vi "QTrkTest.vi"() -> ()   [LabVIEW 2011]
uses:
  QTrk.llb/QTrkSettings.ctl
panel:
  in  "Select dll":bool
  out "Sample img":sgl[][](graph)
  in  "stop test":bool
  out "Frame#":i32
  out "Frames/s":dbl
  in  "Testing sample count":i32=10000
  out "testing results":i32
  out "Single ZLUT plane image":sgl[][](graph)
  in  "Run":bool
  in  "stop":bool
  in  "LUT radii":cluster{"min":sgl, "max":sgl}={"min"=0.0, "max"=40.0}
  out "LUT":u8[][](graph)
  out "zlut results":i32
  out "Generated LUT":sgl[][](graph)
  in  "Max Z":dbl=180.0
  in  "Min Z":dbl
  in  "QTrk Settings":T1={"Image width"=150, "Image height"=150, "Number of threads (CPU based)"=-1, "Max Queue Size"=128, "XCOR Profile Length"=32, "XCOR Profile Width"=2, "XCOR Iterations"=5, "ZLUT MinRadius"=5.0, "ZLUT MaxRadius"=60.0, "ZLUT AngularSteps"=128, "QI Iterations"=4, "QI RadialSteps"=64, "QI AngularSteps Per Quadrant"=32, "QI MinRadius"=2.0, "QI MaxRadius"=60.0, "CUDA Device# (if using cuda)"=0, "COM Background correction factor"=2.0, "ZLUT RadialSteps"=64, "Gaussian 2D Fit Iterations"=8}
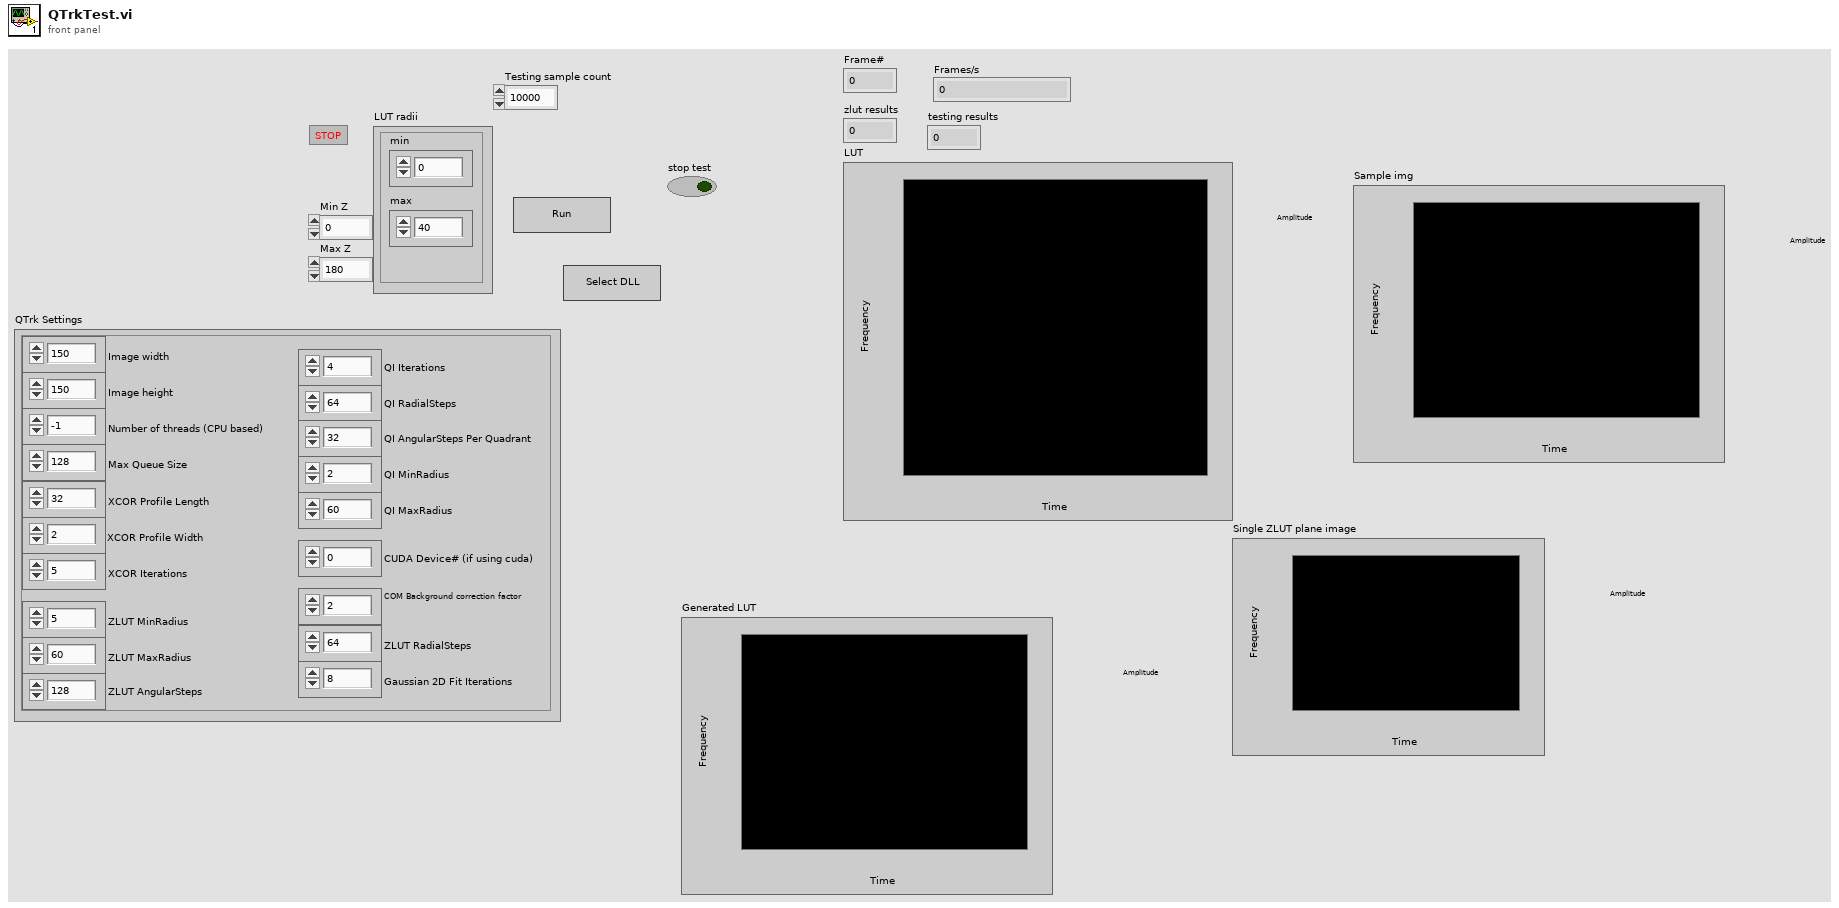
[diagram p1: front panel]
types:
  T1 = typedef "QTrkSettings.ctl" = cluster{"Image width":i32, "Image height":i32, "Number of threads (CPU based)":i32, "Max Queue Size":i32, "XCOR Profile Length":i32, "XCOR Profile Width":i32, "XCOR Iterations":i32, "ZLUT MinRadius":sgl, "ZLUT MaxRadius":sgl, "ZLUT AngularSteps":i32, "QI Iterations":i32, "QI RadialSteps":i32, "QI AngularSteps Per Quadrant":i32, "QI MinRadius":sgl, "QI MaxRadius":sgl, "CUDA Device# (if using cuda)":i32, "COM Background correction factor":sgl, "ZLUT RadialSteps":i32, "Gaussian 2D Fit Iterations":i32}
  T2 = typedef "Image Type" = u32
  T3 = typedef "IMAQ Image.ctl" = refnum<image>
  T4 = enum16{"Center-of-Mass", "1D Cross-Correlation", "Quadrant Interpolation"}
  T5 = typedef "QTrkInstance.ctl" = cluster{"QTrk Pointer":u64, "QTrk Settings":T1}
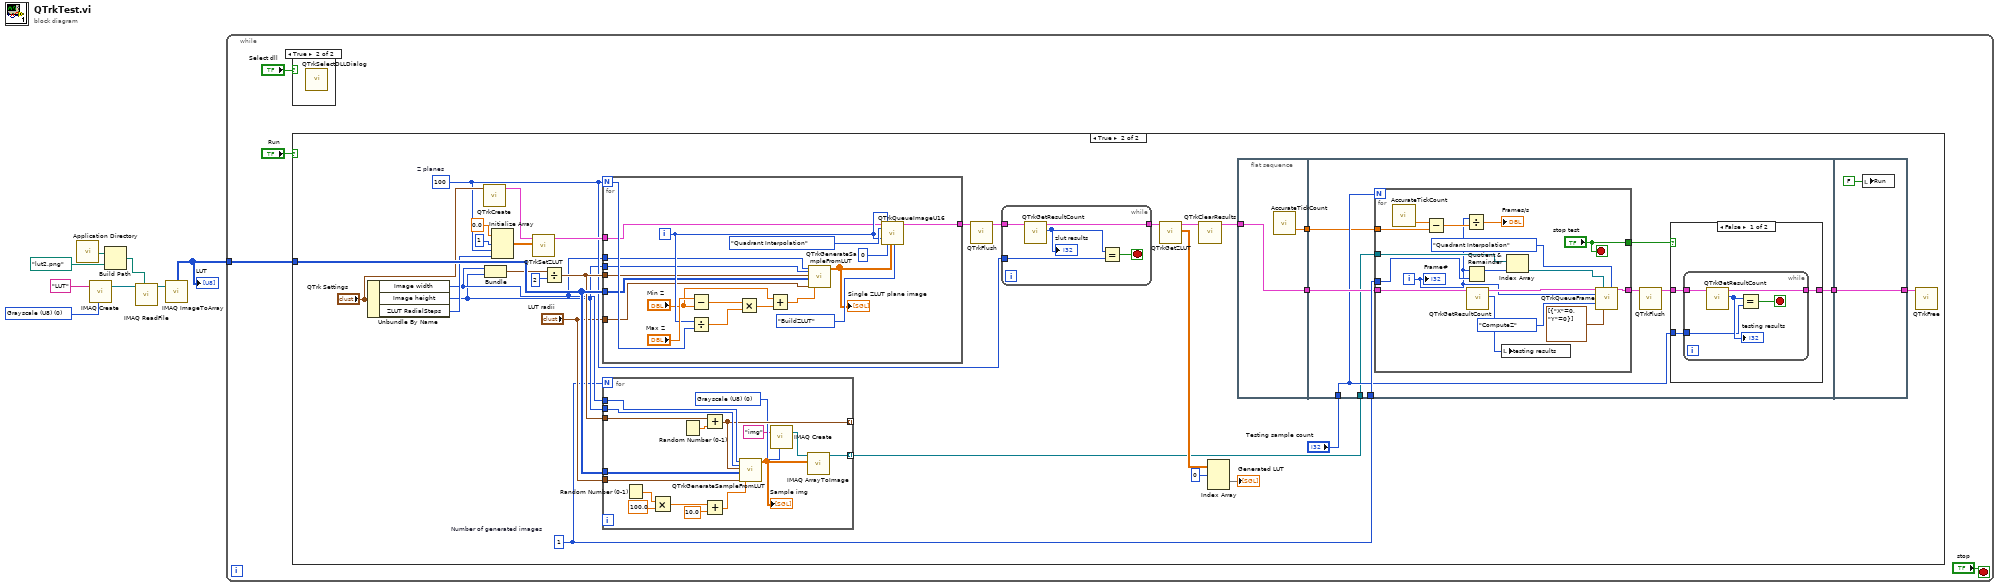
[diagram p0: block diagram]
diagram:
  w8 = T2 0 items=["Grayscale (U8)", "Grayscale (I16)", "Grayscale (SGL)", "Complex (CSG)", "RGB (U32)", "HSL (U32)", "RGB (U64)", "Grayscale (U16)"] ("Image Type")
  n1 = call <vilib>:"Application Directory.vi"() -> ("Application Directory"=w4:path)
  n2 = call "IMAQ Create"("Image Name"="LUT" ("String"), "Image Type"=w8) -> ("New Image"=w6:T3)  [unwired: 3 in, 1 out]
  n3 = Build Path(base path=w4, name or relative path=path "lut2.png" ("File Path")) -> (appended path=w2:path)
  n4 = call "IMAQ ReadFile"("File Path"=w2, "Image"=w6) -> ("Image Out"=w5:T3)  [unwired: 5 in, 4 out]
  n5 = call "IMAQ ImageToArray"("Image"=w5) -> ("Image Pixels (U8)"=w1:u8[][])  [unwired: 3 in, 4 out]
  "LUT" <- w1
  n6 = while {
    tunnel: w1 -> [w12]
    stop <- "stop" stop-if-true
    n7 = case shown="True" "Select dll" {
      frame False {
      }
      frame True {
        n8 = call "QTrkSelectDLLDialog.vi"() -> ()  [unwired: 11 in, 1 out]
      }
    }
    n9 = case shown="True" "Run" {
      tunnel: w12 -> [_ w39]
      frame False {
      }
      frame True {
        w25 = 100  # Z planes
        w20 = 1  # Number of generated images
        n10 = Unbundle By Name("QTrk Settings") -> ("Image width"=w24:i32, "Image height"=w23:i32, "ZLUT RadialSteps"=w32:i32)
        n11 = call "QTrkCreate.vi"("QTrk Settings"="QTrk Settings") -> ("QTrk Instance"=w22:T5)  [unwired: 5 in, 1 out]
        n12 = Bundle("Image width"=w24, "Image height"=w23) -> (w37:cluster{"Image width":i32, "Image height":i32})  [unwired: 1 in]
        n13 = Initialize Array(sgl 0.0 ("element"), 1 ("dimension size"), w25, w32) -> (w35:sgl[][][])
        n14 = call "QTrkSetZLUT.vi"("ZLUT"=w35, "QTrk Instance"=w22) -> ("QTrk Instance"=w30:T5)  [unwired: 8 in, 1 out]
        n15 = Divide(x=w37, y=2 ("Image height")) -> (x/y=w31:cluster{"Image width":dbl, "Image height":dbl})
        n16 = for {
          N: w25 -> [w104]
          tunnel: w31 -> [w95]
          tunnel: w30 -> [w92]
          tunnel: [w98] -> w15
          tunnel: w24 -> [w97]
          tunnel: w23 -> [w96]
          tunnel: w39 -> [w94]
          tunnel: "LUT radii" -> [w93]
          i -> [w100]
          n17 = Subtract(x="Max Z", y="Min Z") -> (x-y=w103:dbl)
          n18 = Divide(x=w100, y=w104) -> (x/y=w102:dbl)
          n19 = Multiply(x=w103, y=w102) -> (x*y=w88:dbl)
          n20 = Add(x="Min Z", y=w88) -> (x+y=w87:dbl)
          n21 = call "QTrkGenerateSampleFromLUT.vi"("Width"=w97, "Height"=w96, "position"=w95, "LUT"=w94, "LUT radii"=w93, "z"=w87) -> ("image"=w90:sgl[][])  [unwired: 13 in]
          "Single ZLUT plane image" <- w90
          n22 = call "QTrkQueueImageU16.vi"("QTrk Instance"=w92, "2D Localization Type"=T4."Quadrant Interpolation", "frame#"=w100, "zlutPlane"=w100, "zlutIndex"=0, "Image (U16)"=w90, "Z Command"=enum16{"Nothing", "ComputeZ", "BuildZLUT"}."BuildZLUT") -> ("QTrk Instance"=w98:T5)  [unwired: 11 in, 1 out]
        }
        n23 = for {
          N: w20 -> [_]
          tunnel: w31 -> [w122]
          tunnel: [w117] -> _ mode=indexing
          tunnel: w24 -> [w119]
          tunnel: w23 -> [w118]
          tunnel: w39 -> [w116]
          tunnel: "LUT radii" -> [w115]
          tunnel: [w108] -> w13 mode=indexing
          w110 = T2 0 items=["Grayscale (U8)", "Grayscale (I16)", "Grayscale (SGL)", "Complex (CSG)", "RGB (U32)", "HSL (U32)", "RGB (U64)", "Grayscale (U16)"] ("Image Type")
          n24 = Random Number (0-1)() -> (number: 0 to 1=w113:dbl)
          n25 = Multiply(x=w113, y=100.0) -> (x*y=w111:dbl)
          n26 = Random Number (0-1)() -> (number: 0 to 1=w121:dbl)
          n27 = Add(x=w122, y=w121) -> (x+y=w117:cluster{"Image width":dbl, "Image height":dbl})
          n28 = Add(x=w111, y=10.0) -> (x+y=w114:dbl)
          n29 = call "QTrkGenerateSampleFromLUT.vi"("Width"=w119, "Height"=w118, "position"=w117, "LUT"=w116, "LUT radii"=w115, "z"=w114) -> ("image"=w107:sgl[][])  [unwired: 13 in]
          "Sample img" <- w107
          n30 = call "IMAQ Create"("Image Name"="img", "Image Type"=w110) -> ("New Image"=w109:T3)  [unwired: 3 in, 1 out]
          n31 = call "IMAQ ArrayToImage"("Image Pixels (U8)"=w107, "Image"=w109) -> ("Image Out"=w108:T3)  [unwired: 8 in, 1 out]
        }
        n32 = call "QTrkFlush.vi"("QTrk Instance"=w15) -> ("QTrk Instance (out)"=w14:T5)  [unwired: 9 in, 1 out]
        n33 = while {
          tunnel: w14 -> [w86]
          tunnel: [w85] -> w26
          tunnel: w25 -> [w83]
          stop <- w82 stop-if-true
          n34 = call "QTrkGetResultCount.vi"("QTrk Instance"=w86) -> ("result count"=w84:i32, "QTrk Instance"=w85:T5)  [unwired: 4 in, 1 out]
          "zlut results" <- w84
          n35 = Equal?(x=w84, y=w83) -> (x = y?=w82:bool)
        }
        n36 = call "QTrkGetZLUT.vi"("QTrk Instance (in)"=w26) -> ("zlut"=w29:sgl[][][], "QTrk Instance"=w17:T5)  [unwired: 8 in, 1 out]
        n37 = call "QTrkClearResults.vi"("QTrk Instance (in)"=w17) -> ("QTrk Instance (out)"=w16:T5)  [unwired: 10 in]
        n38 = Index Array(array=w29, index (dim 0)=0 ("index (page)")) -> (element=→"Generated LUT":sgl[][])  [unwired: 2 in]
        n39 = flat-sequence {
          tunnel: w16 -> [w44]
          tunnel: [w44] -> w42
          tunnel: [w43] -> w41
          tunnel: w20 -> [w53]
          tunnel: "Testing sample count" -> [w50]
          tunnel: w42 -> [w51]
          tunnel: [w52] -> w40
          tunnel: w41 -> [w48]
          tunnel: w13 -> [w45]
          tunnel: [w81] -> w18
          tunnel: w40 -> [w81]
          frame #0 {
            n40 = call "AccurateTickCount.vi"() -> ("seconds"=w43:dbl)  [unwired: 2 in, 1 out]
          }
          frame #1 {
            n41 = for {
              N: w50 -> [_]
              tunnel: w51 -> [w77]
              tunnel: w53 -> [w79]
              tunnel: [w63] -> w47
              tunnel: ["stop test"] -> w49
              tunnel: w48 -> [w72]
              tunnel: w45 -> [w70]
              i -> [w67]
              stop <- "stop test" stop-if-true
              n42 = call "AccurateTickCount.vi"() -> ("seconds"=w71:dbl)  [unwired: 2 in, 1 out]
              n43 = Subtract(x=w71, y=w72) -> (x-y=w73:dbl)
              n44 = Divide(x=w67, y=w73) -> (x/y=→"Frames/s":dbl)
              n45 = Quotient & Remainder(x=w67, y=w79) -> (x-y*floor(x/y)=w78:i32)  [unwired: 1 out]
              n46 = call "QTrkGetResultCount.vi"("QTrk Instance"=w77) -> ("result count"=w76:i32, "QTrk Instance"=w69:T5)  [unwired: 4 in, 1 out]
              n47 = local write "testing results"(w76) -> ()
              n48 = Index Array(array=w70, index=w78) -> (element=w68:T3)
              n49 = call "QTrkQueueFrame.vi"("QTrk Instance"=w69, "Image"=w68, "2D Localization Type"=T4."Quadrant Interpolation", "frame#"=w67, "Z Command"=enum16{"Nothing", "ComputeZ", "BuildZLUT"}."ComputeZ", "ROI Positions (corner-based)"=cluster{"X":i32, "Y":i32}[] [{"X"=0, "Y"=0}]) -> ("QTrk Instance (out)"=w63:T5)  [unwired: 8 in, 1 out]
              "Frame#" <- w67
            }
            n50 = call "QTrkFlush.vi"("QTrk Instance"=w47) -> ("QTrk Instance (out)"=w46:T5)  [unwired: 9 in, 1 out]
            n51 = case shown="False" w49 {
              tunnel: w46 -> [w56 w62]
              tunnel: [w55 w62] -> w52
              tunnel: w50 -> [w54 _]
              frame False {
                n52 = while {
                  tunnel: w56 -> [w57]
                  tunnel: [w61] -> w55
                  tunnel: w54 -> [w59]
                  stop <- w58 stop-if-true
                  n53 = call "QTrkGetResultCount.vi"("QTrk Instance"=w57) -> ("result count"=w60:i32, "QTrk Instance"=w61:T5)  [unwired: 4 in, 1 out]
                  "testing results" <- w60
                  n54 = Equal?(x=w60, y=w59) -> (x = y?=w58:bool)
                }
              }
              frame True {
              }
            }
          }
          frame #2 {
            n55 = local write "Run"(FALSE ("Run")) -> ()
          }
        }
        n56 = call "QTrkFree.vi"("QTrk Instance"=w18) -> ()  [unwired: 6 in, 1 out]
      }
    }
  }
